vi "ELVIS III v1.0 Close UART.vi"(8 "error in (no error)":errorcluster, 11 "VISA resource name in":refnum<visa-resource-name>) -> (0 "error out":errorcluster)   [LabVIEW 2021]
uses:
  <vilib>/myRIO/Common/Instrument Driver Framework/Utilities/typedefs/FPGA Ref Manager Action Enum.ctl
  <vilib>/myRIO/Common/Instrument Driver Framework/ELVIS III v1.0/UART/vis/ELVIS III v1.0 Build MUX Configuration UART.vi
  <vilib>/myRIO/Common/Instrument Driver Framework/ELVIS III v1.0/UART/vis/ELVIS III v1.0 Configure UART.vi
  <vilib>/myRIO/Common/Instrument Driver Framework/ELVIS III v1.0/Resource Manager/vis/ELVIS III v1.0 Unreserve Channel List.vi
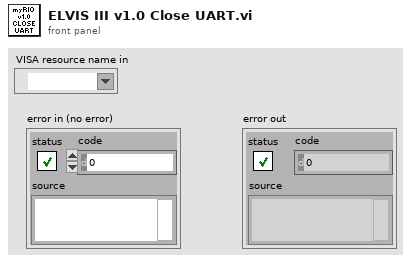
[diagram p1: front panel]
types:
  T1 = typedef "FPGA Ref Manager Action Enum.ctl" = enum16{"Get", "Set", "Reset"}
  T2 = typedef "Generic FPGA Reference.ctl" = refnum<k20>
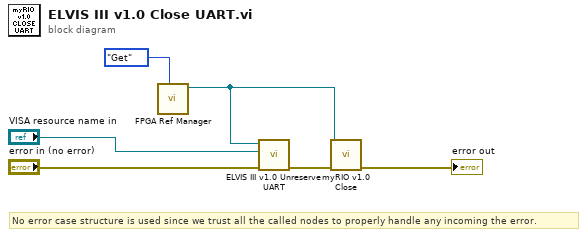
[diagram p0: block diagram]
diagram:
  # "No error case structure is used since we trust all the called nodes to properly handle any incoming the error."
  n1 = call <vilib>:"FPGA Ref Manager.vi"("Action"=FPGA_Ref_Manager_Action_Enum."Get") -> ("Generic FPGA Reference out"=w1:T2)  [unwired: 8 in, 1 out]
  n2 = call <vilib>:"ELVIS III v1.0 Unreserve UART.vi"("error in (no error)"="error in (no error)", "VISA resource name in"="VISA resource name in", "myRIO FPGA Ref In"=w1) -> ("error out"=w6:errorcluster)  [unwired: 8 in]
  n3 = call <vilib>:"myRIO v1.0 Close.vi"("error in (no error)"=w6, "myRIO FPGA Ref In"=w1) -> ("error out"=→"error out":errorcluster)  [unwired: 9 in]
